vi "getTokenElement.vi"(7 "Endpoint Element Name":string, 8 "error in (no error)":errorcluster, 10 "Token element":T1, 11 "Oauth2 in":refnum<class "Oauth2.lvclass">) -> (0 "error out":errorcluster, 1 "Value":string, 2 "Key":string, 3 "Oauth2 out":refnum<class "Oauth2.lvclass">)   [LabVIEW 2013, in "Oauth2.lvclass"]
uses:
  Oauth2.lvclass
  OAuthToken/OAuth2 Token Element -- enum.ctl
  Oauth2.lvclass/Oauth2.ctl
  OAuthToken/OAuthAccessToken.lvclass
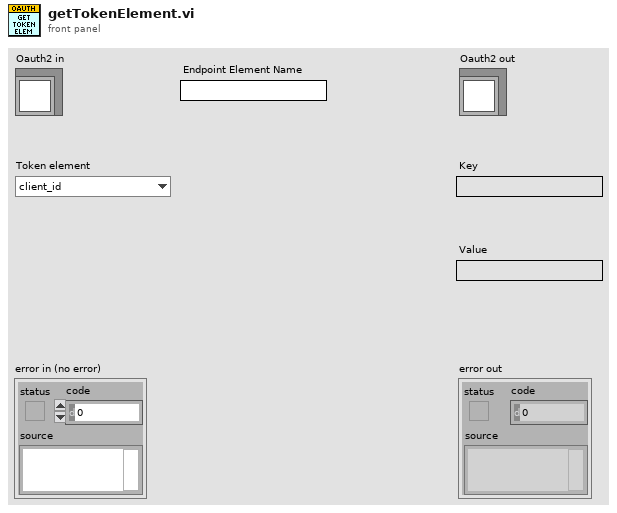
[diagram p1: front panel]
types:
  T1 = typedef "OAuthAccessToken.lvclass/OAuth2 Token Element -- enum.ctl" = enum16{"client_id", "client_secret", "response_type", "scope", "redirect_uri", "error", "error_description", "error_uri", "grant_type", "code", "access_token", "token_type", "expires_in", "username", "password", "refresh_token", "endpoint element"}
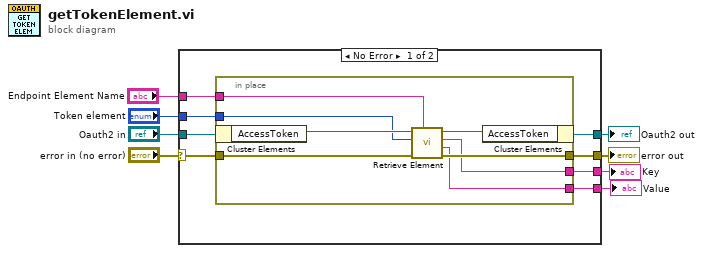
[diagram p0: block diagram]
diagram:
  n1 = case shown="No Error" "error in (no error)" {
    selector: "error in (no error)" -> [w14 w26]
    tunnel: [w13 w26] -> w7
    tunnel: [w15 w25] -> w5
    tunnel: "Oauth2 in" -> [w16 w25]
    tunnel: "Token element" -> [w12 _]
    tunnel: "Endpoint Element Name" -> [w11 _]
    tunnel: [w10 _] -> w2
    tunnel: [w9 _] -> w1
    frame No Error {
      n2 = in-place {
        in-place-border: w14 -> [w21]
        in-place-border: [w20] -> w13
        in-place-border: w12 -> [w22]
        in-place-border: w11 -> [w24]
        in-place-border: [w18] -> w10
        in-place-border: [w17] -> w9
        n3 = in-place-cluster #1(w16) -> ("AccessToken"=w23:refnum<class "OAuthAccessToken.lvclass">)
        n4 = call "Retrieve Element.vi"("Endpoint element key"=w24, "error in (no error)"=w21, "Token element"=w22, "OAuthAccessToken in"=w23) -> ("error out"=w20:errorcluster, "Value"=w17:string, "Key"=w18:string, "OAuthAccessToken out"=w19:refnum<class "OAuthAccessToken.lvclass">)  [unwired: 4 in]
        n5 = in-place-cluster #1("AccessToken"=w19) -> (w15:refnum<class "Oauth2.lvclass">)
      }
    }
    frame Error {
    }
  }
  "error out" <- w7
  "Oauth2 out" <- w5
  "Value" <- w1
  "Key" <- w2
